vi "Pcre2GetOvectorCount8.vi"(8 "error in":errorcluster, 11 "pMatchData":u64 format="%.0x") -> (0 "error out":errorcluster, 2 "OvectorCount":u32, 3 "pMatchData":u64 format="%.0x")   [LabVIEW 2021, in "libpcre2-8.lvlib"]
uses:
  libpcre2-8.lvlib
  libpcre2-8-x32.dll
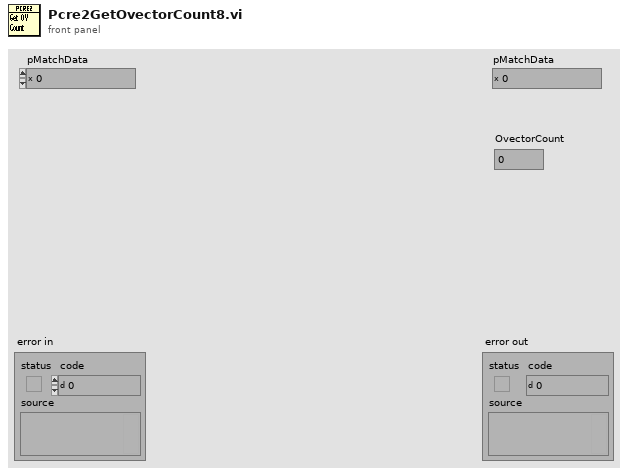
[diagram p1: front panel]
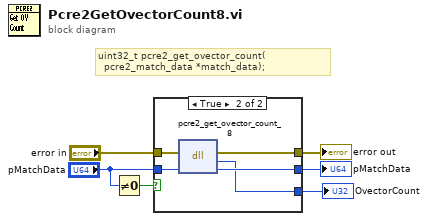
[diagram p0: block diagram]
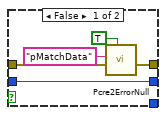
[diagram p2: hidden frame]
diagram:
  # "uint32_t pcre2_get_ovector_count(\n  pcre2_match_data *match_data);"
  n1 = Not Equal To 0?(x="pMatchData") -> (x != 0?=w2:bool)
  n2 = case shown="True" w2 {
    tunnel: "error in" -> [w9 w13]
    tunnel: [w11 w16] -> w5
    tunnel: [w10 w14] -> w4
    tunnel: [_ w12] -> w1
    tunnel: "pMatchData" -> [w11 w15]
    frame False {
      n3 = call "Pcre2ErrorNull.vi"("IsPointer? (F)"=TRUE, "error in"=w9, "What"="pMatchData") -> ("error out"=w10:errorcluster)  [unwired: 8 in]
    }
    frame True {
      n4 = dll-call lib="libpcre2-8-x*.dll" fn="pcre2_get_ovector_count_8"(error in=w13, "match_data"=w15) -> (error out=w14:errorcluster, "OvectorCount"=w12:u32, "match_data"=w16:u64)  [unwired: 2 in, 1 out]
    }
  }
  "pMatchData" <- w5
  "error out" <- w4
  "OvectorCount" <- w1
